vi "Root Actor.vi"(6 "Unified Actor Alias":string, 9 "Core Leaf Actors":refnum<class "Actor.lvclass">[](array[class]), 10 "Actors":refnum<class "Actor.lvclass">[](array[class])) -> (0 "Error out":errorcluster, 2 "Root Unified Actor DVR":refnum<data-value>)   [LabVIEW 2020, in "jettl.lvlib" / "Spawn.lvlib"]
uses:
  Spawn.lvlib
  jettl.lvlib
  Unified Actor.ctl
  Unified Actor Lifetime.ctl
  Msg/Msg.lvclass
  Msg Set.ctl
  Unified Actor Relation.ctl
  Teller.ctl
  Msg Contents/Msg Contents.lvclass
  Msg.ctl
  Actor/Actor.lvclass
  Msgs.ctl
  Base jettl Actor/Base jettl Actor.lvlib
  Base jettl Actor/Init Actor.vi
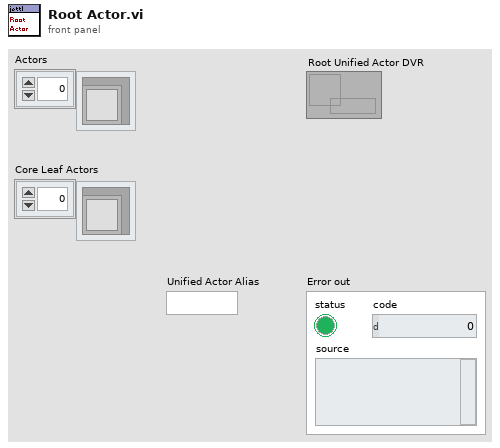
[diagram p1: front panel]
types:
  T1 = typedef "jettl.lvlib/Msgs.ctl" = cluster{"Inbound":T2, "Outbound":T2, "Implemented":T2, "Tell Init":T2, "Tell Init Self":T2, "Tell Init Parent":T2, "Tell Init Child":T2, "Tell Forward":T2, "Tell Forward Self":T2, "Tell Forward Parent":T2, "Tell Forward Child":T2}
  T2 = typedef "jettl.lvlib/Msg Set.ctl" = set{refnum<class "Msg.lvclass">}
  T3 = typedef "jettl.lvlib/Unified Actor.ctl" = cluster{"Msgs":T1, "Leaf":bool, "Edge Actors":refnum<class "Actor.lvclass">[], "Mid Actors":refnum<class "Actor.lvclass">[], "Core Actors":refnum<class "Actor.lvclass">[], "Root":bool, "Alias":string, "Transport":refnum<user-event>, "Address":refnum<event-registration>, "This VI":refnum<vi>}
  T4 = typedef "jettl.lvlib/Unified Actor Lifetime.ctl" = enum16{"Init", "Spawn", "Setup", "Teardown Before Running", "Running", "Stop Called", "Stopping With Children", "Stopping Without Children", "Teardown After Running", "Stopped"}
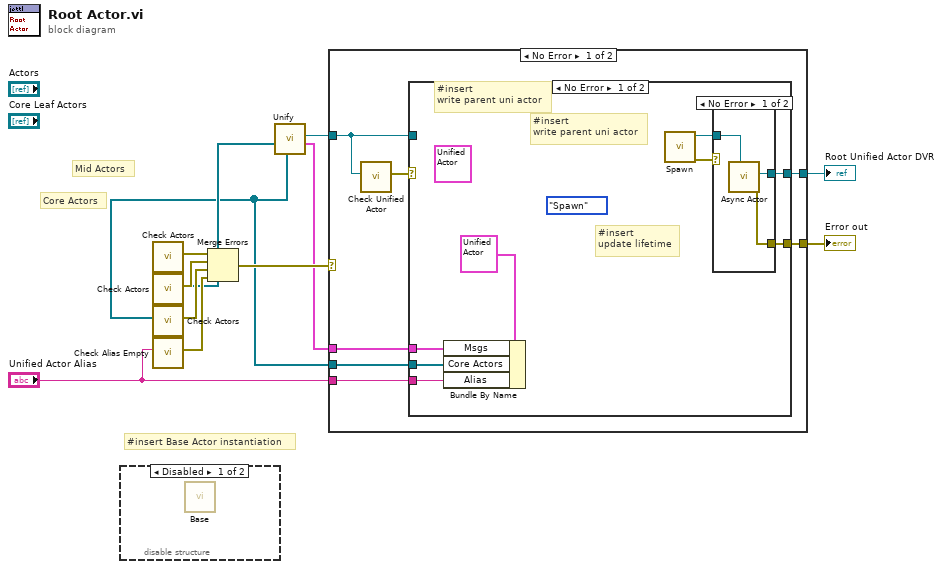
[diagram p0: block diagram]
diagram:
  # "Core Actors"
  # "Mid Actors"
  # "#insert Base Actor instantiation"
  n1 = disable-structure shown="Disabled" {
    frame Disabled {
      n2 = call-poly "Base.vi"() -> ()  [unwired: 11 in, 1 out]
    }
    frame Enabled {
    }
  }
  n3 = call "Check Actors.vi"() -> ("Error"=w7:errorcluster)  [unwired: 11 in]
  n4 = call "Check Actors.vi"() -> ("Error"=w11:errorcluster, "Actors"=w6:refnum<class "Actor.lvclass">[])  [unwired: 10 in]
  n5 = call "Check Actors.vi"() -> ("Error"=w8:errorcluster, "Actors"=w5:refnum<class "Actor.lvclass">[])  [unwired: 10 in]
  n6 = call "Check Alias Empty.vi"("Alias"="Unified Actor Alias") -> ("Error"=w10:errorcluster)  [unwired: 10 in]
  n7 = Merge Errors(w7, w11, w8, w10) -> (w12:errorcluster)
  n8 = call "Unify.vi"("Core Actors"=w5, "Mid Actors"=w6) -> ("Msgs"=w3:T1, "Unified Actor"=w2:refnum<class "Actor.lvclass">)  [unwired: 7 in, 1 out]
  n9 = case shown="No Error" w12 {
    selector: w12 -> [_ w37]
    tunnel: [w19 w37] -> w1
    tunnel: [w18 _] -> w4
    tunnel: "Unified Actor Alias" -> [w17 _]
    tunnel: w5 -> [w13 _]
    tunnel: w3 -> [w15 _]
    tunnel: w2 -> [w14 _]
    frame No Error {
      n10 = call "Check Unified Actor.vi"("Unified Actor"=w14) -> ("Error"=w16:errorcluster)  [unwired: 10 in]
      n11 = case shown="No Error" w16 {
        selector: w16 -> [_ w36]
        tunnel: [w31 w36] -> w19
        tunnel: [w30 _] -> w18
        tunnel: w17 -> [w29 _]
        tunnel: w15 -> [w27 _]
        tunnel: w14 -> [w22 _]
        tunnel: w13 -> [w23 _]
        frame No Error {
          w21 = Unified_Actor_Lifetime."Spawn" ("Lifetime")
          (unwired) T3 {"Msgs"={"Inbound"={}, "Outbound"={}, "Implemented"={}, "Tell Init"={}, "Tell Init Self"={}, "Tell Init Parent"={}, "Tell Init Child"={}, "Tell Forward"={}, "Tell Forward Self"={}, "Tell Forward Parent"={}, "Tell Forward Child"={}}, "Leaf"=FALSE, "Edge Actors"=[], "Mid Actors"=[], "Core Actors"=[], "Root"=FALSE, "Alias"="", "Transport"=refnum, "Address"=refnum, "This VI"=refnum} ("Parent Actor Attributes")
          # "#insert\nupdate lifetime"
          # "#insert\nwrite parent uni actor"
          # "#insert\nwrite parent uni actor"
          n12 = Bundle By Name(cluster=T3 {"Msgs"={"Inbound"={}, "Outbound"={}, "Implemented"={}, "Tell Init"={}, "Tell Init Self"={}, "Tell Init Parent"={}, "Tell Init Child"={}, "Tell Forward"={}, "Tell Forward Self"={}, "Tell Forward Parent"={}, "Tell Forward Child"={}}, "Leaf"=FALSE, "Edge Actors"=[], "Mid Actors"=[], "Core Actors"=[], "Root"=FALSE, "Alias"="", "Transport"=refnum, "Address"=refnum, "This VI"=refnum} ("Attributes"), "Msgs"=w27, "Core Actors"=w23, "Alias"=w29) -> (w26:T3)
          n13 = call-dynamic "Spawn.vi"() -> ("Error out"=w24:errorcluster, "Actor out"=w25:refnum<class "Actor.lvclass">, "Actor in"=w20:refnum<class "Actor.lvclass">)  [unwired: 9 in]
          n14 = case shown="No Error" w24 {
            selector: w24 -> [_ w35]
            tunnel: [w34 w35] -> w31
            tunnel: [w33 _] -> w30
            tunnel: w25 -> [w32 _]
            frame No Error {
              n15 = call "Async Actor.vi"("Actor in"=w32) -> ("Error out"=w34:errorcluster, "Child Unified Actor DVR"=w33:refnum<data-value>)  [unwired: 9 in]
            }
            frame Error {
            }
          }
        }
        frame Error {
        }
      }
    }
    frame Error {
    }
  }
  "Error out" <- w1
  "Root Unified Actor DVR" <- w4
